vi "JKI_UI Console.vi"() -> ()   [LabVIEW 2017, in "UI Console_JKI.lvlib"]
uses:
  UI Console_JKI.lvlib
  <userlib>/_NEVSTOP/JKI State Machine ++/_Support/_Create Data Queue.vi
  <userlib>/_NEVSTOP/JKI State Machine ++/_Support/_JKISMQFGV.vi
  <userlib>/_NEVSTOP/JKI State Machine ++/JKI-State-Machine-Plus.lvlib
panel:
  in  "Error Simulator":bool
  in  "Transaction Enable Signal":bool
  in  "KeyPad Enable Signal":bool
  in  "Keypad":T1
  out "Keypad String":string
  in  "Card Reader Enable Signal":bool
  in  "Transactions":T2
  in  "Card Reader":bool
  out "State History":string
  in  "Name(\"\" to use uuid)":string="UI Console"
  # "KeyPad"
  # "Transaction"
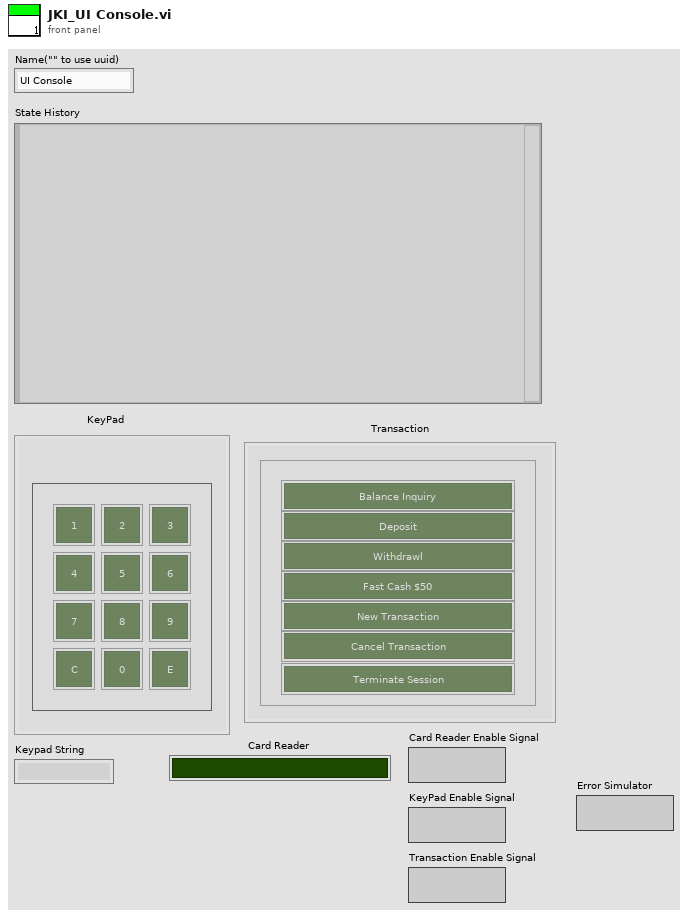
[diagram p1: front panel]
types:
  T1 = cluster{"Key":bool, "Key 2":bool, "Key 3":bool, "Key 4":bool, "Key 5":bool, "Key 6":bool, "Key 7":bool, "Key 8":bool, "Key 9":bool, "Key 10":bool, "Key 11":bool, "Key 12":bool}
  T2 = cluster{"xaction":bool, "xaction 2":bool, "xaction 3":bool, "xaction 4":bool, "xaction 5":bool, "xaction 6":bool, "xaction 7":bool}
  T3 = enum32{"Invalid", "Standard", "Closed", "Hidden", "Minimized", "Maximized"}
  T4 = enum32{"invalid app kind", "Development System", "Run Time System", "Student Edition", "Embedded LabVIEW", "Evaluation", "Custom"}
  T5 = enum8{"Enabled", "Disabled", "Disabled and Grayed Out"}
  T6 = cluster{"Core":cluster{"Current VI Reference":refnum<vi>, "Close Panel on Exit?":bool}, "Your Boolean data":bool, "New Character":i32, "Keypad String":string, "Transaction Type":i32}
  T7 = cluster{"Current VI Reference":refnum<vi>, "Close Panel on Exit?":bool}
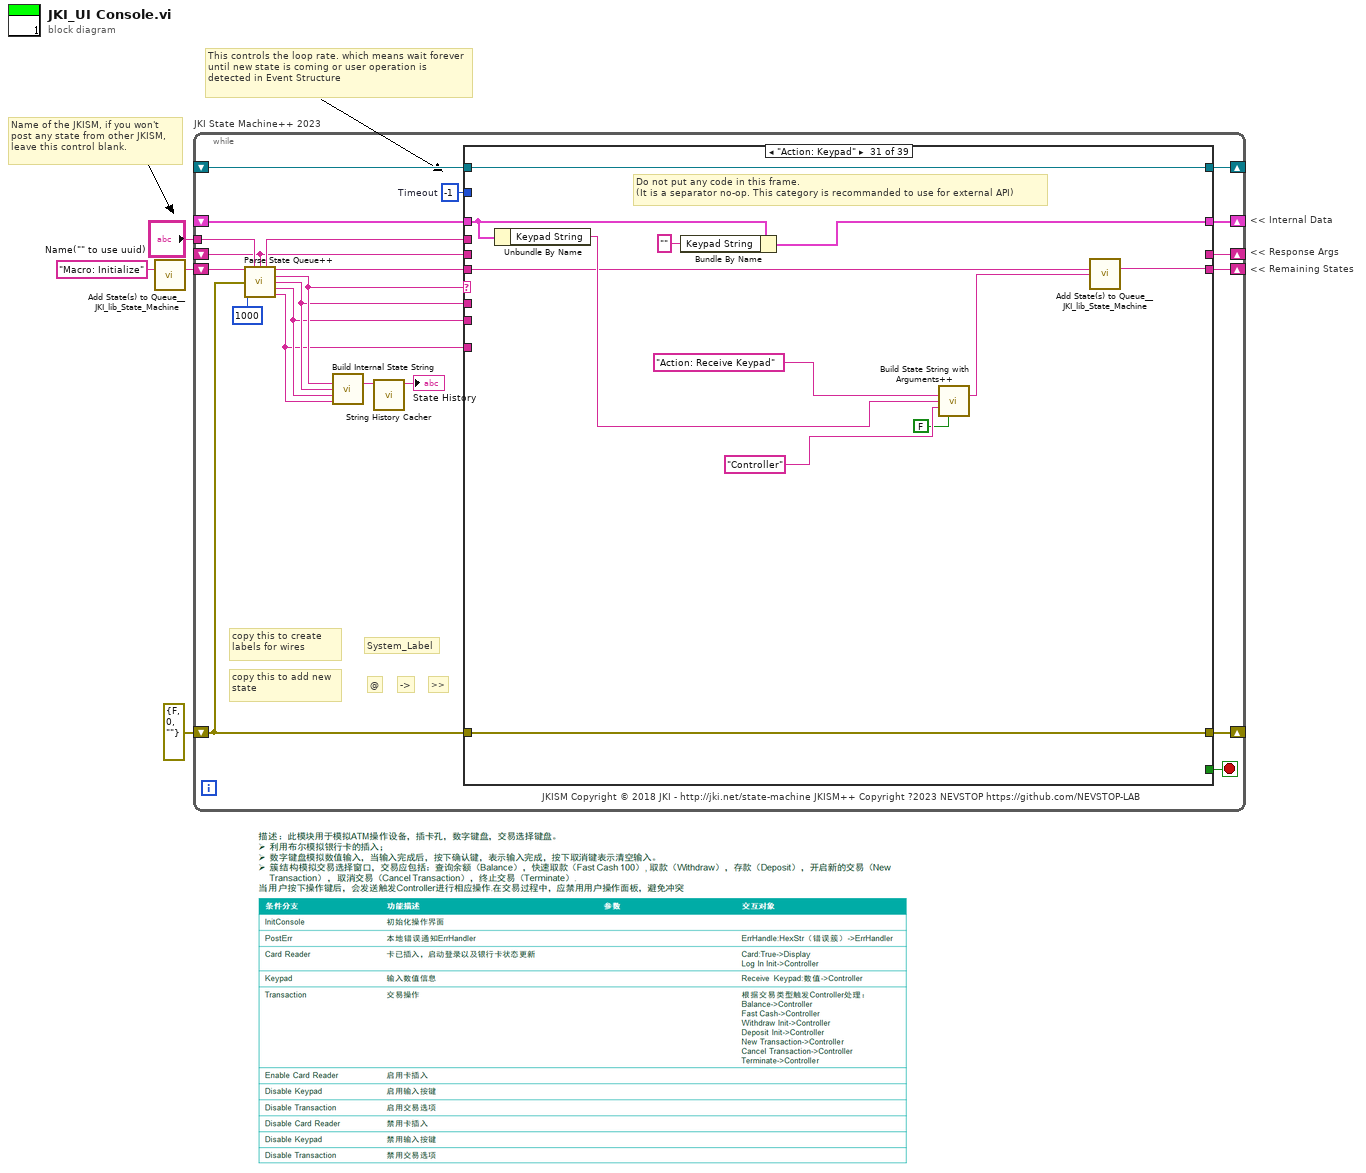
[diagram p0: block diagram]
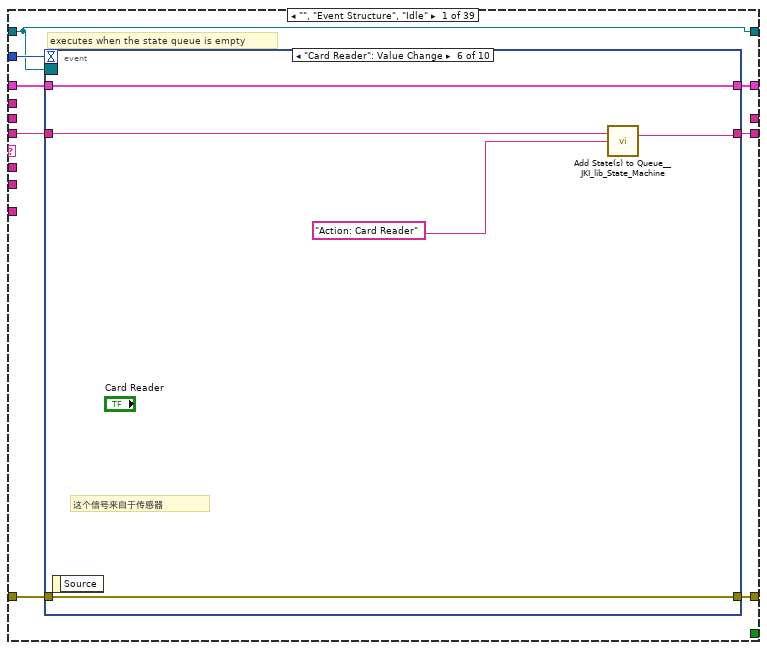
[diagram p2: hidden frame]
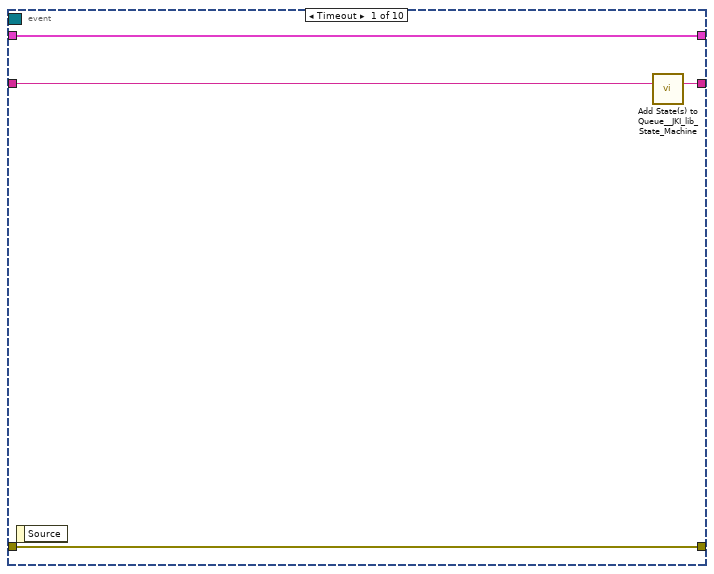
[diagram p3: hidden frame]
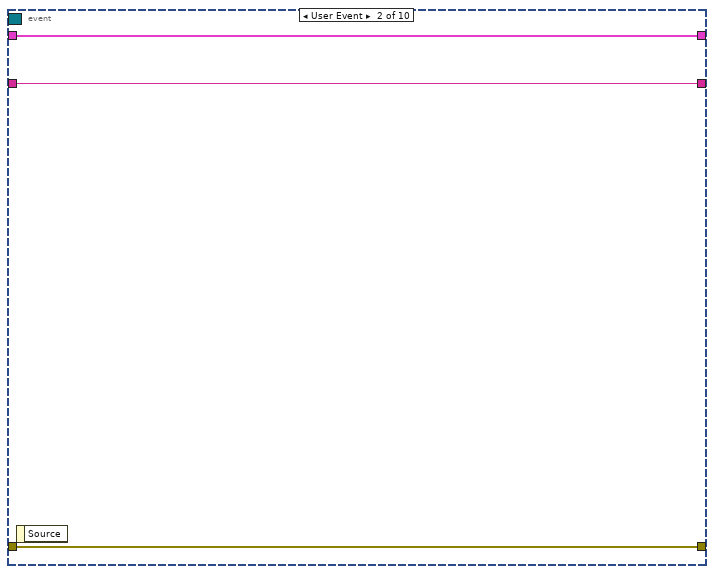
[diagram p4: hidden frame]
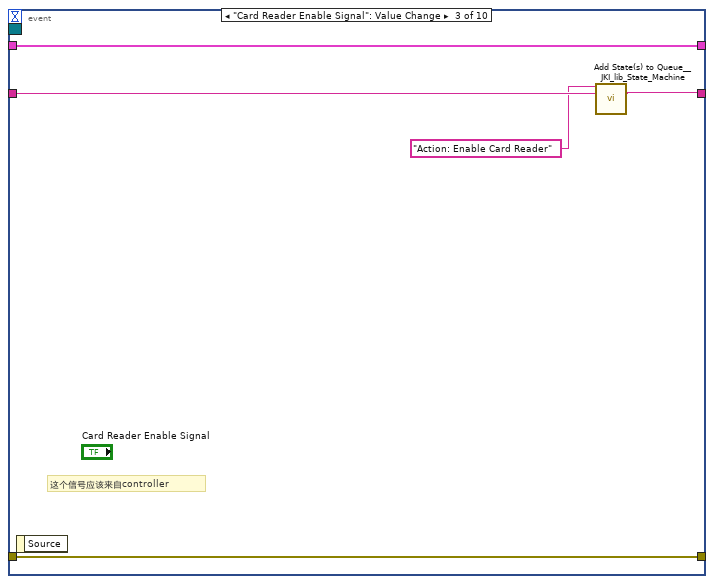
[diagram p5: hidden frame]
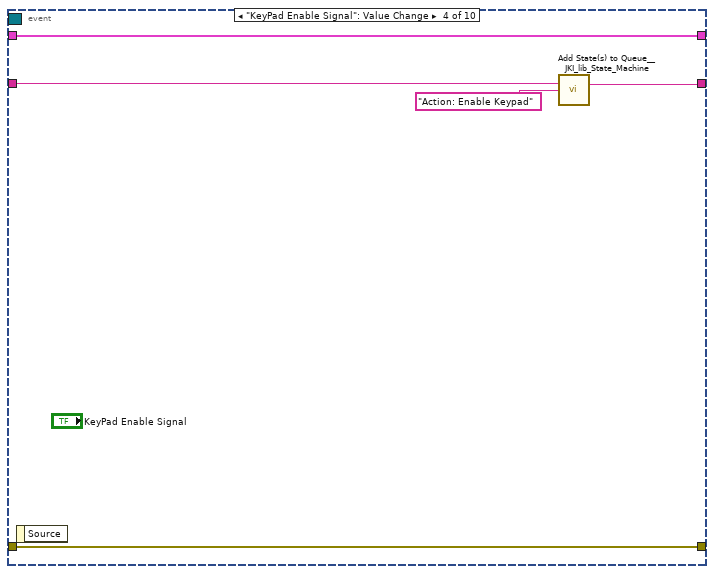
[diagram p6: hidden frame]
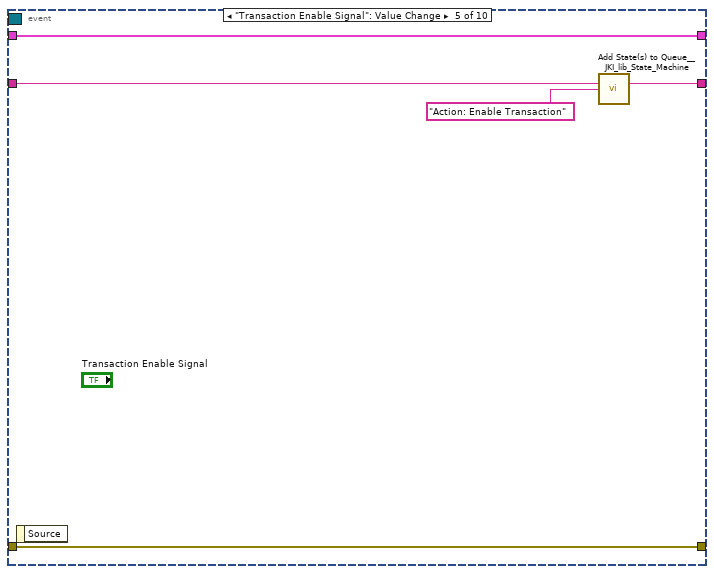
[diagram p7: hidden frame]
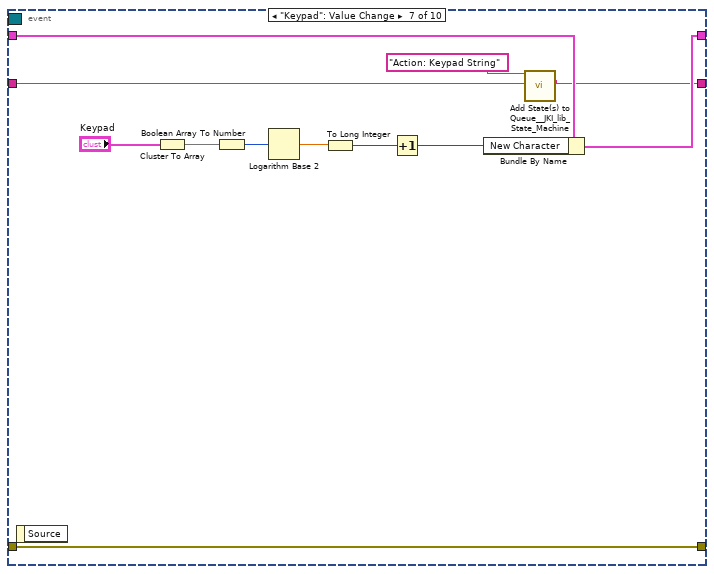
[diagram p8: hidden frame]
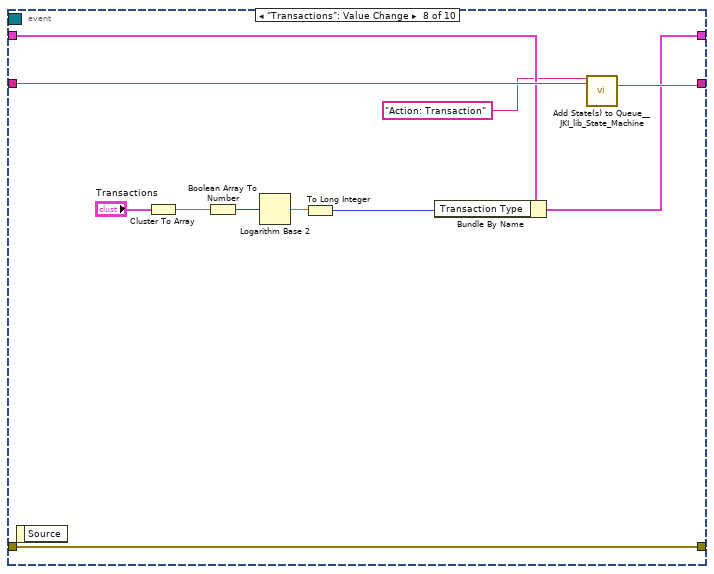
[diagram p9: hidden frame]
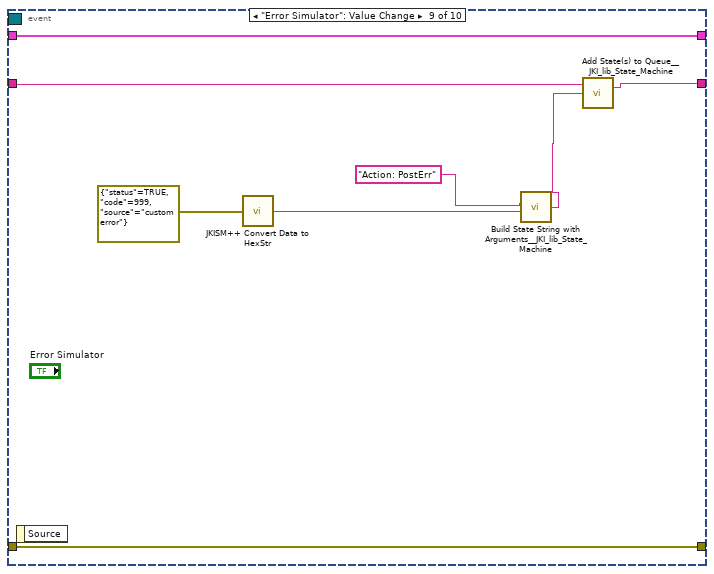
[diagram p10: hidden frame]
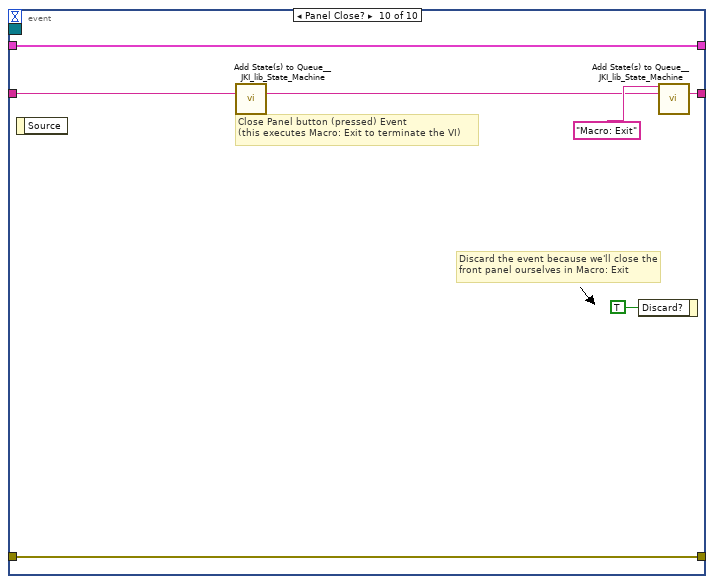
[diagram p11: hidden frame]
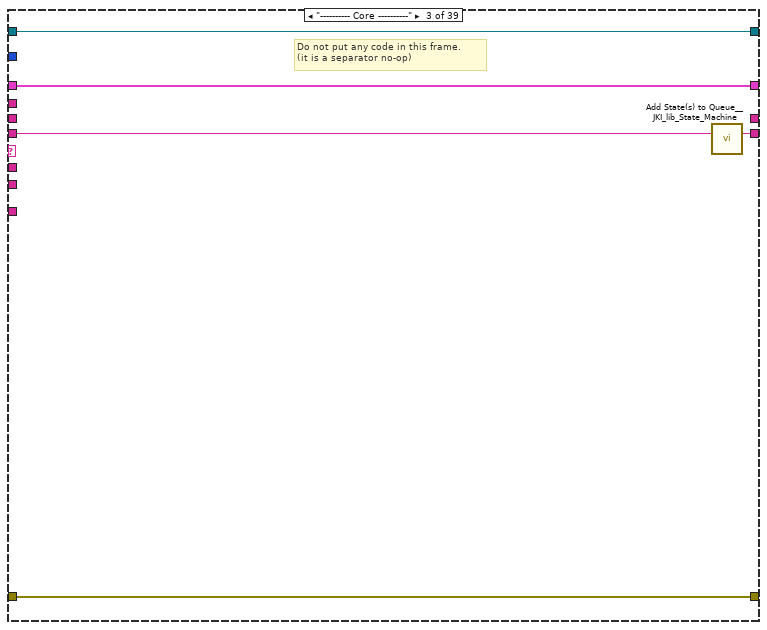
[diagram p13: hidden frame]
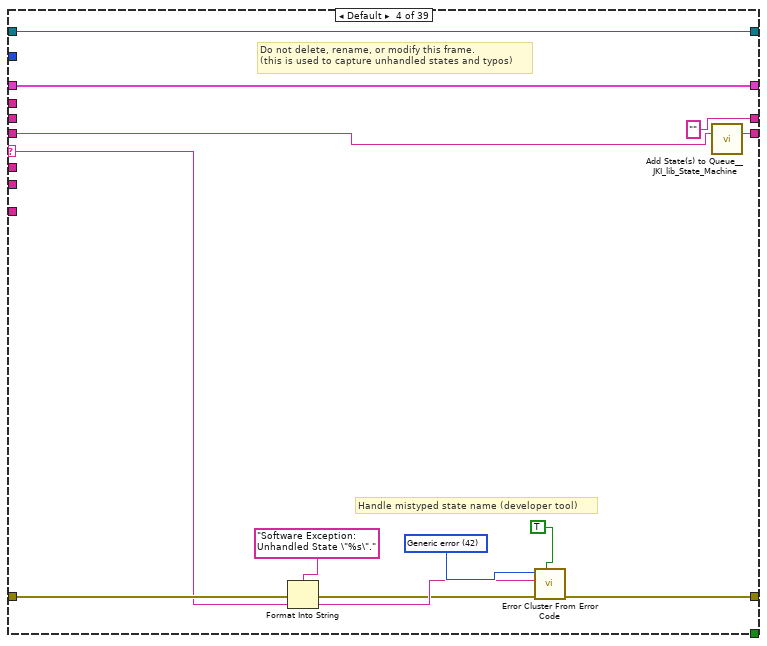
[diagram p14: hidden frame]
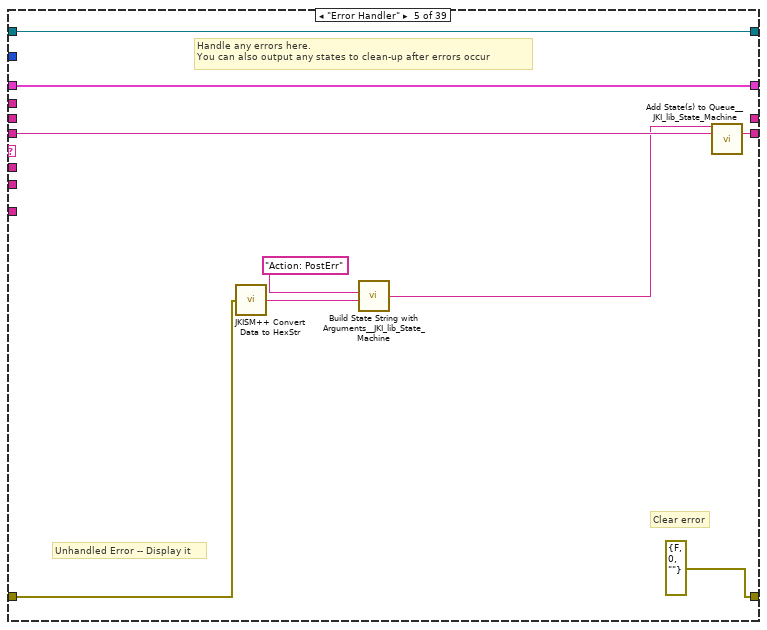
[diagram p15: hidden frame]
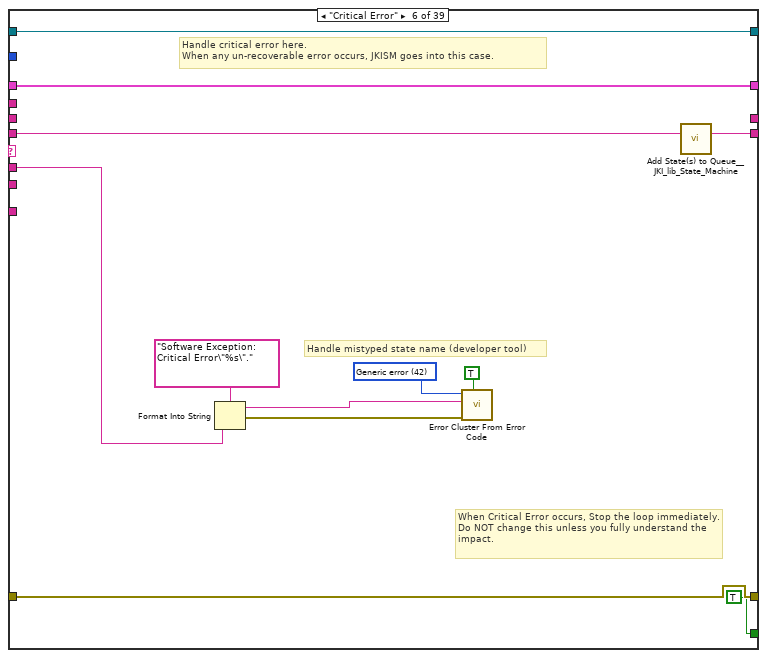
[diagram p16: hidden frame]
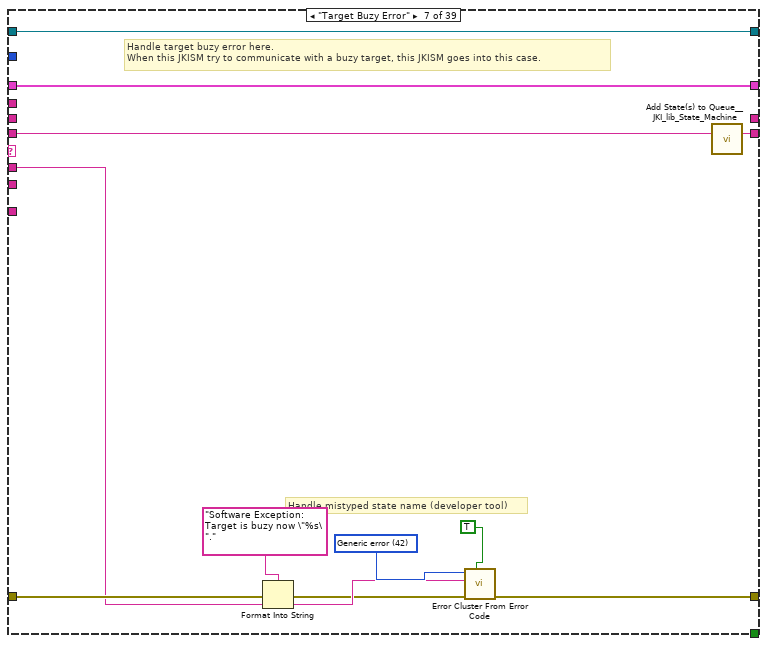
[diagram p17: hidden frame]
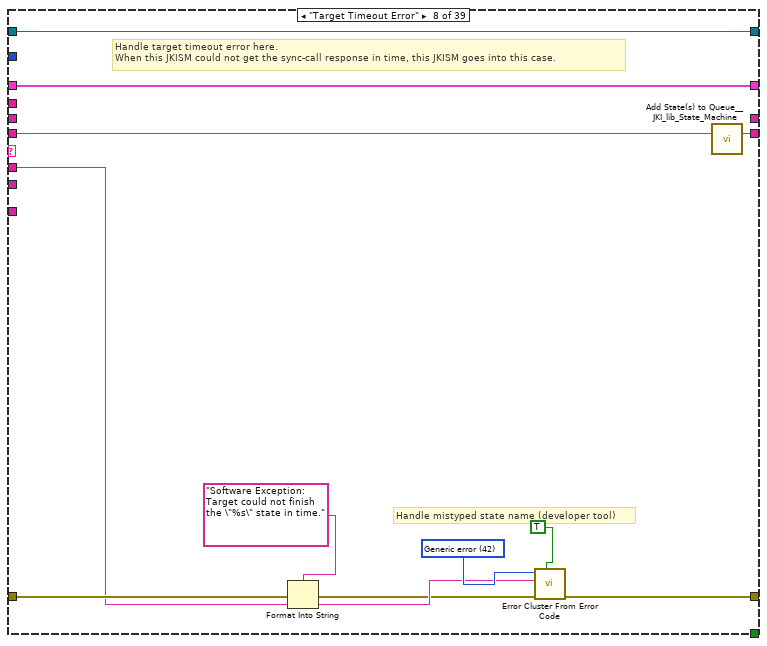
[diagram p18: hidden frame]
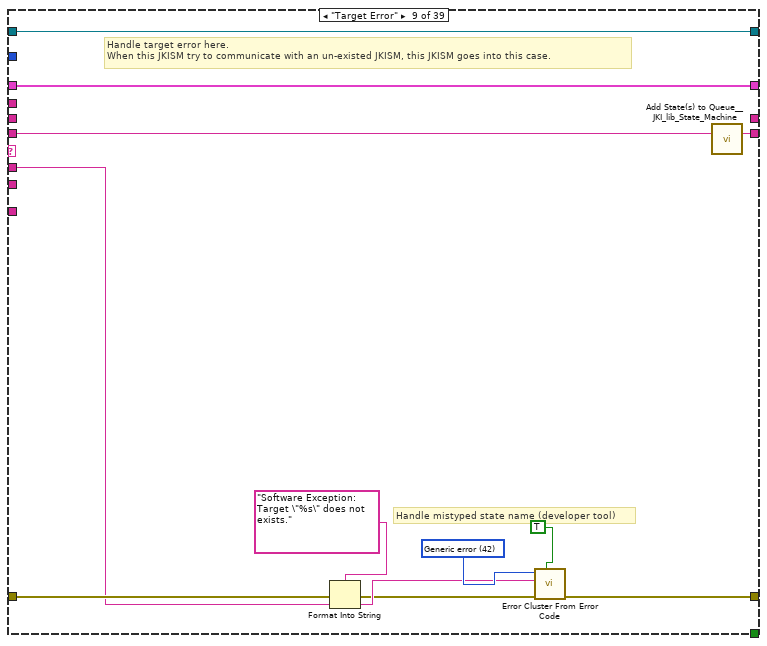
[diagram p19: hidden frame]
diagram:
  # "<< Internal Data"
  # "<< Response Args"
  # "<< Remaining States"
  # "Name of the JKISM, if you won't post any state from other JKISM,  leave this control blank."
  # "This controls the loop rate. which means wait forever until new state is coming or user operation is detected in Event Structure"
  n1 = call <vilib>:"Add State(s) to Queue__JKI_lib_State_Machine.vi"("State(s) in (\"\")"="Macro: Initialize") -> ("States Out"=w2:string)  [unwired: 14 in]
  n2 = while "JKI State Machine++ 2023" {
    shift-right: [w21] -> _
    shift-left: _ -> [w20]
    shift-right: [w24] -> _
    shift-left: errorcluster {"status"=FALSE, "code"=0, "source"=""} ("error out") -> [w18]
    shift-right: [w23] -> _
    shift-left: w2 -> [w25]
    tunnel: "Name(\"\" to use uuid)" -> [w13]
    shift-right: [w16] -> _
    shift-left: _ -> [w5]
    shift-right: [w15] -> _
    shift-left: _ -> [w14]
    stop <- w22 stop-if-true
    w19 = -1  # Timeout
    # "JKISM Copyright © 2018 JKI - http://jki.net/state-machine JKISM++ Copyright ?2023 NEVSTOP https://github.com/NEVSTOP-LAB"
    # "copy this to add new state"
    # ">>"
    # "->"
    # "@"
    # "copy this to create labels for wires"
    # "System_Label"
    n3 = call <userlib>:"Parse State Queue++.vi"("State Queue"=w25, "Name(\"\" to use uuid)"=w13, "Response Arguments"=w5, "Error In (no error)"=w18, "Response Timeout(5000ms)"=1000 ("Response Timeout(1000ms)")) -> ("Name Used"=w6:string, "Remaining States"=w26:string, "Current State"=w10:string, "Arguments"=w9:string, "Argument - State"=w8:string, "From Who"=w7:string)  [unwired: 5 in]
    n4 = call <userlib>:"Build Internal State String.vi"("State"=w10, "Arguments (\"\")"=w9, "Arg-State (\"\")"=w8, "Source (\"\")"=w7) -> ("State with Arguments"=w11:string)  [unwired: 11 in]
    n5 = call <userlib>:"String History Cacher.vi"("String"=w11) -> ("String Cache"=→"State History":string)  [unwired: 10 in]
    n6 = case shown="\"Action: Keypad\"" w10 {
      selector: w10 -> [_ _ _ w111 _ _ _ _ _ _ _ _ _ _ _ _ _ _ _ _ _ _ _ _ _ _ _ _ _ _ _ _ _ _ _ _ _ _ _]
      tunnel: w26 -> [w34 w102 w108 w115 w130 w140 w143 w160 w172 w181 w185 w200 w206 w211 w221 w228 w233 w239 w243 w249 w254 w261 w273 w343 w349 w360 w365 w377 w385 w401 w420 w430 w471 w491 w498 w505 w512 w519 w526]
      tunnel: w9 -> [_ _ _ _ _ w133 w145 w156 w168 _ _ _ _ _ _ _ _ _ _ _ _ w256 w267 _ _ _ _ _ w381 _ _ _ _ _ _ _ _ _ _]
      tunnel: w20 -> [w32 w101 w105 w113 w127 w141 w147 w158 w170 w180 w184 w193 w204 w208 _ w223 w230 w238 w242 w246 w252 w259 w269 w340 w346 w357 w362 w375 w387 w414 w417 w432 w465 w489 w496 w503 w510 w517 w524]
      tunnel: [w31 w103 w106 w117 errorcluster {"status"=FALSE, "code"=0, "source"=""} ("error out") w142 w150 w162 w174 w182 w186 w197 w203 w209 w218 w224 w231 w234 w241 w247 w251 w257 w270 w341 w347 w358 w363 w369 w379 w407 w425 w427 w469 w485 w492 w499 w506 w513 w520] -> w24
      tunnel: w18 -> [w30 w103 w106 w116 w123 w142 w149 w161 w173 w182 w186 w197 w203 w209 w218 w225 w231 _ w244 w247 w251 w258 w271 w341 w347 w358 w363 w367 w380 w407 w425 w427 w469 w486 w493 w500 w507 w514 w521]
      tunnel: [w33 w102 w107 w114 w129 w139 w148 w159 w171 w181 w185 w199 w205 w210 w220 w227 w232 w239 w243 w248 w253 w260 w272 w342 w348 w359 w364 w376 w384 w400 w419 w429 w470 w490 w497 w504 w511 w518 w525] -> w23
      tunnel: [_ _ _ _ _ TRUE _ _ _ _ _ _ TRUE _ _ _ _ _ _ _ _ _ _ _ _ _ _ _ _ _ _ _ _ _ _ _ _ _ _] -> w22
      tunnel: [w29 w101 w105 w113 w127 w141 w147 w158 w170 w180 w184 w198 w204 w208 w219 w223 w230 w238 w242 w246 w252 w259 w269 w340 w346 w357 w362 w375 w387 w414 w415 w432 w464 w489 w496 w503 w510 w517 w524] -> w21
      tunnel: w19 -> [w28 _ _ _ _ _ _ _ _ _ _ _ _ _ _ _ _ _ _ _ _ _ _ _ _ _ _ _ _ _ _ _ _ _ _ _ _ _ _]
      tunnel: w7 -> [_ _ _ _ _ _ _ _ _ _ _ _ _ _ _ _ _ _ _ _ _ _ _ _ _ _ _ _ _ _ _ _ _ _ _ _ _ _ _]
      tunnel: w8 -> [_ _ _ _ _ _ _ _ _ _ _ _ _ _ _ _ _ _ _ _ _ _ _ _ _ _ _ _ _ _ _ _ _ _ _ _ _ _ _]
      tunnel: [_ _ _ "" _ _ _ _ _ _ _ _ _ _ _ _ _ _ _ _ _ _ _ _ _ _ _ _ _ _ _ _ w462 _ _ _ _ _ _] -> w16
      tunnel: [w27 w100 w104 w109 w126 w131 w144 w155 w167 w179 w183 w187 w201 w207 w215 w222 w229 w237 w240 w245 w250 w255 w266 w339 w344 w350 w361 w374 w386 w413 w426 w433 w468 w488 w495 w502 w509 w516 w523] -> w15
      tunnel: w14 -> [w27 w100 w104 w109 w126 w131 w144 w155 w167 w179 w183 w187 w201 w207 w215 w222 w229 _ w240 w245 w250 w255 w266 w339 w344 w350 w361 w374 w386 w413 w426 w433 w468 w488 w495 w502 w509 w516 w523]
      tunnel: w6 -> [_ _ _ _ _ _ _ _ _ _ _ _ _ _ _ _ _ w236 _ _ _ _ _ _ _ _ _ _ _ _ _ _ _ _ _ _ _ _ _]
      tunnel: w5 -> [_ _ _ _ _ _ _ _ _ _ _ _ _ _ _ _ _ _ _ _ _ _ _ _ _ _ _ _ _ _ _ _ _ _ _ _ _ _ _]
      frame "", "Event Structure", "Idle" {
        # "executes when the state queue is empty"
        n7 = event shown="[5] \"Card Reader\": Value Change" {
          selector: w27 -> [_ _ _ _ _ _ _ _ _ _]
          dyn-events: _ -> [_ _ _ _ _ _ _ _ _ _]
          timeout: w28 -> [_ _ _ _ _ _ _ _ _ _]
          tunnel: w34 -> [w38 w41 w45 w49 w54 w59 w68 w79 w87 w93]
          tunnel: [w37 w41 w44 w48 w53 w58 w67 w78 w86 w99] -> w33
          tunnel: w32 -> [w35 w39 w46 w50 w55 w61 w71 w77 w91 w97]
          tunnel: [w36 w40 w43 w51 w56 w60 w73 w84 w92 w98] -> w31
          tunnel: w30 -> [w36 w40 w43 w51 w56 w60 w73 w84 w92 w98]
          tunnel: [w35 w39 w46 w50 w55 w61 w70 w75 w91 w97] -> w29
          event Timeout {
            n8 = event-data() -> ()  [unwired: 1 in, 1 out]
            n9 = call <vilib>:"Add State(s) to Queue__JKI_lib_State_Machine.vi"("State(s) in (\"\")"=w38) -> ("States Out"=w37:string)  [unwired: 14 in]
          }
          event User Event {
            n10 = event-data() -> ()  [unwired: 1 in, 1 out]
          }
          event "Card Reader Enable Signal": Value Change {
            # "这个信号应该来自controller"
            n11 = event-data() -> ()  [unwired: 1 in, 1 out]
            n12 = call <vilib>:"Add State(s) to Queue__JKI_lib_State_Machine.vi"("State(s) in Front (\"\")"="Action: Enable Card Reader", "State(s) in (\"\")"=w45) -> ("States Out"=w44:string)  [unwired: 13 in]
          }
          event "KeyPad Enable Signal": Value Change {
            n13 = event-data() -> ()  [unwired: 1 in, 1 out]
            n14 = call <vilib>:"Add State(s) to Queue__JKI_lib_State_Machine.vi"("State(s) in (\"\")"=w49, "State(s) at Back (\"\")"="Action: Enable Keypad" ("State(s) at Back (\"\")")) -> ("States Out"=w48:string)  [unwired: 13 in]
          }
          event "Transaction Enable Signal": Value Change {
            n15 = event-data() -> ()  [unwired: 1 in, 1 out]
            n16 = call <vilib>:"Add State(s) to Queue__JKI_lib_State_Machine.vi"("State(s) in (\"\")"=w54, "State(s) at Back (\"\")"="Action: Enable Transaction" ("State(s) at Back (\"\")")) -> ("States Out"=w53:string)  [unwired: 13 in]
          }
          event "Card Reader": Value Change {
            # "这个信号来自于传感器"
            n17 = event-data() -> ()  [unwired: 1 in, 1 out]
            n18 = call <vilib>:"Add State(s) to Queue__JKI_lib_State_Machine.vi"("State(s) in (\"\")"=w59, "State(s) at Back (\"\")"="Action: Card Reader") -> ("States Out"=w58:string)  [unwired: 13 in]
          }
          event "Keypad": Value Change {
            n19 = event-data() -> ()  [unwired: 1 in, 1 out]
            n20 = Cluster To Array(cluster="Keypad") -> (array=w64:bool[])
            n21 = Boolean Array To Number(Boolean array=w64) -> (number=w72:u32)
            n22 = Logarithm Base 2(1:w72) -> (0:w69:dbl)
            n23 = To Long Integer(number=w69) -> (32bit integer=w63:i32)
            n24 = Increment(x=w63) -> (x+1=w62:i32)
            n25 = Bundle By Name(cluster=w71, "New Character"=w62) -> (w70:T6)
            n26 = call <vilib>:"Add State(s) to Queue__JKI_lib_State_Machine.vi"("State(s) in Front (\"\")"="Action: Keypad String" ("State(s) in Front (\"\")"), "State(s) in (\"\")"=w68) -> ("States Out"=w67:string)  [unwired: 13 in]
          }
          event "Transactions": Value Change {
            n27 = event-data() -> ()  [unwired: 1 in, 1 out]
            n28 = Cluster To Array(cluster="Transactions") -> (array=w81:bool[])
            n29 = Boolean Array To Number(Boolean array=w81) -> (number=w83:u32)
            n30 = Logarithm Base 2(1:w83) -> (0:w82:dbl)
            n31 = To Long Integer(number=w82) -> (32bit integer=w76:i32)
            n32 = Bundle By Name(cluster=w77, "Transaction Type"=w76) -> (w75:T6)
            n33 = call <vilib>:"Add State(s) to Queue__JKI_lib_State_Machine.vi"("State(s) in Front (\"\")"="Action: Transaction" ("State(s) in Front (\"\")"), "State(s) in (\"\")"=w79) -> ("States Out"=w78:string)  [unwired: 13 in]
          }
          event "Error Simulator": Value Change {
            n34 = event-data() -> ()  [unwired: 1 in, 1 out]
            n35 = call <userlib>:"JKISM++ Convert Data to HexStr.vi"("Variant"=errorcluster {"status"=TRUE, "code"=999, "source"="custom error"} ("error in (no error)")) -> ("HEX String (0-9,A-F)"=w89:string)  [unwired: 8 in]
            n36 = call <vilib>:"Build State String with Arguments__JKI_lib_State_Machine.vi"("Arguments (\"\")"=w89, "State"="Action: PostErr" ("States")) -> ("State with Arguments"=w88:string)  [unwired: 4 in]
            n37 = call <vilib>:"Add State(s) to Queue__JKI_lib_State_Machine.vi"("State(s) in (\"\")"=w87, "State(s) at Back (\"\")"=w88) -> ("States Out"=w86:string)  [unwired: 13 in]
          }
          event Panel Close? {
            # "Discard the event because we'll close the front panel ourselves in Macro: Exit"
            # "Close Panel button (pressed) Event\n(this executes Macro: Exit to terminate the VI)"
            n38 = event-data() -> ()  [unwired: 1 in, 1 out]
            n39 = call <vilib>:"Add State(s) to Queue__JKI_lib_State_Machine.vi"("State(s) in (\"\")"=w93) -> ("States Out"=w94:string)  [unwired: 14 in]
            n40 = event-data("Discard?"=TRUE) -> ()  [unwired: 1 in, 1 out]
            n41 = call <vilib>:"Add State(s) to Queue__JKI_lib_State_Machine.vi"("State(s) in Front (\"\")"="Macro: Exit", "State(s) in (\"\")"=w94) -> ("States Out"=w99:string)  [unwired: 13 in]
          }
        }
      }
      frame "JKISM++ Documentation" {
        # "JKISM++ Documentation"
        # "State Syntax:\nStateCategory: State >> Argument @|-> JKISMName\nLine Terminator: Line feed\n\nExample:\nUI: Help >> About @Main\nUI: Help >> About ->Main"
        # "Commenting:\nTo add a comment use \"//\" or \"#\" and all text to the right will be ignored\nCommenting Example:\nUI: Initialize // This initializes the UI\n# This whole line is a comment\n// Another comment line"
        # "Where \"UI\" is the state category\nWhere \"Help\" is the state\nWhere \"About\" is the argument\nWhere \"Main\" is the Name of JKISM,which actually run the \"UI: Help >> About\"\n\n    \"@\" stands for sync state. Current JKISM will wait until the state is finished. \n            - if \"Main\" named JKISM does not exist, \"Target Error\" will occur.\n            - if \"Main\" named JKISM is in another sync remote state, \"Target Buzy Error\" will occur.\n            - if \"Main\" named JKISM could not finish the state in time, \"Target Timeout Error\" will occur.\n            - if everything is right. \"Response\" will occur with Argument back from \"Main\" named JKISM. \n\n    \"->\" stands for async state. Current JKISM will post the state and continue to next state in next iteration.\n            - if \"Main\" named JKISM does not exist, \"Target Error\" will occur.\n            - if everything is right. \"Async Message Posted\" will occur.\n            - After State is finished. Caller will receive a \"Async Response\" state from callee.\n\nWhen duplicated name is used for multiple JKISM module or some framework problem happens, \"Critical Error\" will occur."
      }
      frame "---------- Core ----------" {
        # "Do not put any code in this frame.\n(it is a separator no-op)"
        n42 = call <vilib>:"Add State(s) to Queue__JKI_lib_State_Machine.vi"("State(s) in (\"\")"=w108) -> ("States Out"=w107:string)  [unwired: 14 in]
      }
      frame Default {
        w120 = 42 items=["No error", "Argument error", "Memory is full", "Out of zone", "End of file", "File already open", "Generic file I/O error", "File not found", "File permission error", "Disk is full", "Duplicate path", "Too many files open", "System feature not enabled", "Resource file not found", "Cannot add resource", "Resource not found", "Image not found", "Image memory error", "Pen does not exist", "Config type invalid", "Config token not found", "Config parse error", "Config memory error", "Bad external code format", "Bad external code offset", "External code not present", "Null window", "Destroy window error", "Null menu", "Print aborted", "Bad print record", "Print driver error", "Windows error during printing", "Memory error during printing", "Print dialog error", "Generic print error", "Invalid device refnum", "Device not found", "Device parameter error", "Device unit error", "Cannot open device", "Device call aborted", "Generic error", "Cancelled by user", "Object ID too low", "Object ID too high", "Object not in heap", "Unknown heap", "Unknown object (invalid DefProc)", "Unknown object (DefProc not in table)", "Message out of range", "Invalid (null) method", "Unknown message", "Manager call not supported", "Bad address", "Network operation in progress", "Network operation timed out", "Connection is busy", "Network attribute not supported", "Network error", "Address in use", "System out of memory", "Connection aborted", "Connection refused", "Not connected", "Already connected", "Connection closed", "Initialization error (interapplication manager)", "Bad occurrence", "Wait on unbound occurrence handler", "Occurrence queue overflow", "Datalog type conflict", "Unused", "Unrecognized type (interapplication manager)", "Memory corrupt", "Failed to make temporary DLL", "Old CIN version", "Drag socket not found", "Failed to load drop-object", "Failed to register OLE object", "Failed to release OLE object", "Format specifier type mismatch", "Unknown format specifier", "Too few format specifiers", "Too many format specifiers", "Scan failed", "Newer CIN version", "Error converting to variant", "Runtime menu error", "Password tampered", "Variant attribute not found", "Incompatible variant data type", "Event data is not available", "Event Store is not present", "Occurrence is not found", "Event Queue is not created", "Event info is not available", "Refnum passed is NULL", "Error retrieving Class GUID", "Error retrieving CoClass GUID", "Error retrieving TypeLib GUID.", "Bad built application magic bytes.", "Specific driver is different from the specific driver associated with the Logical Name.", "There is no session opened to the class driver.", "Max Error", "MAX - Error with config objects", "MAX - Error loading configuration", "MAX - Group not supported"]
        # "Do not delete, rename, or modify this frame.\n(this is used to capture unhandled states and typos)"
        # "Handle mistyped state name (developer tool)"
        n43 = Format Into String(format string="Software Exception: Unhandled State \"%s\"." ("message"), error in=w116, w111) -> (resulting string=w119:string, error out=w118:errorcluster)  [unwired: 1 in]
        n44 = call <vilib>:"Error Cluster From Error Code.vi"("show call chain? (False)"=TRUE, "error in (no error)"=w118, "error message (\"\")"=w119, "error code (0)"=w120) -> ("error out"=w117:errorcluster)  [unwired: 5 in]
        n45 = call <vilib>:"Add State(s) to Queue__JKI_lib_State_Machine.vi"("State(s) in (\"\")"=w115) -> ("States Out"=w114:string)  [unwired: 14 in]
      }
      frame "Error Handler" {
        # "Unhandled Error -- Display it"
        # "Handle any errors here.\nYou can also output any states to clean-up after errors occur"
        # "Clear error"
        n46 = call <userlib>:"JKISM++ Convert Data to HexStr.vi"("Variant"=w123) -> ("HEX String (0-9,A-F)"=w125:string)  [unwired: 8 in]
        n47 = call <vilib>:"Build State String with Arguments__JKI_lib_State_Machine.vi"("Arguments (\"\")"=w125, "State"="Action: PostErr") -> ("State with Arguments"=w122:string)  [unwired: 4 in]
        n48 = call <vilib>:"Add State(s) to Queue__JKI_lib_State_Machine.vi"("State(s) in Front (\"\")"=w122, "State(s) in (\"\")"=w130) -> ("States Out"=w129:string)  [unwired: 13 in]
      }
      frame "Critical Error" {
        w137 = 42 items=["No error", "Argument error", "Memory is full", "Out of zone", "End of file", "File already open", "Generic file I/O error", "File not found", "File permission error", "Disk is full", "Duplicate path", "Too many files open", "System feature not enabled", "Resource file not found", "Cannot add resource", "Resource not found", "Image not found", "Image memory error", "Pen does not exist", "Config type invalid", "Config token not found", "Config parse error", "Config memory error", "Bad external code format", "Bad external code offset", "External code not present", "Null window", "Destroy window error", "Null menu", "Print aborted", "Bad print record", "Print driver error", "Windows error during printing", "Memory error during printing", "Print dialog error", "Generic print error", "Invalid device refnum", "Device not found", "Device parameter error", "Device unit error", "Cannot open device", "Device call aborted", "Generic error", "Cancelled by user", "Object ID too low", "Object ID too high", "Object not in heap", "Unknown heap", "Unknown object (invalid DefProc)", "Unknown object (DefProc not in table)", "Message out of range", "Invalid (null) method", "Unknown message", "Manager call not supported", "Bad address", "Network operation in progress", "Network operation timed out", "Connection is busy", "Network attribute not supported", "Network error", "Address in use", "System out of memory", "Connection aborted", "Connection refused", "Not connected", "Already connected", "Connection closed", "Initialization error (interapplication manager)", "Bad occurrence", "Wait on unbound occurrence handler", "Occurrence queue overflow", "Datalog type conflict", "Unused", "Unrecognized type (interapplication manager)", "Memory corrupt", "Failed to make temporary DLL", "Old CIN version", "Drag socket not found", "Failed to load drop-object", "Failed to register OLE object", "Failed to release OLE object", "Format specifier type mismatch", "Unknown format specifier", "Too few format specifiers", "Too many format specifiers", "Scan failed", "Newer CIN version", "Error converting to variant", "Runtime menu error", "Password tampered", "Variant attribute not found", "Incompatible variant data type", "Event data is not available", "Event Store is not present", "Occurrence is not found", "Event Queue is not created", "Event info is not available", "Refnum passed is NULL", "Error retrieving Class GUID", "Error retrieving CoClass GUID", "Error retrieving TypeLib GUID.", "Bad built application magic bytes.", "Specific driver is different from the specific driver associated with the Logical Name.", "There is no session opened to the class driver.", "Max Error", "MAX - Error with config objects", "MAX - Error loading configuration", "MAX - Group not supported"]
        # "Handle critical error here.\nWhen any un-recoverable error occurs, JKISM goes into this case."
        # "When Critical Error occurs, Stop the loop immediately. Do NOT change this unless you fully understand the impact."
        # "Handle mistyped state name (developer tool)"
        n49 = Format Into String(format string="Software Exception: Critical Error\"%s\"." ("message"), w133) -> (resulting string=w136:string, error out=w135:errorcluster)  [unwired: 2 in]
        n50 = call <vilib>:"Error Cluster From Error Code.vi"("show call chain? (False)"=TRUE, "error in (no error)"=w135, "error message (\"\")"=w136, "error code (0)"=w137) -> ()  [unwired: 5 in, 1 out]
        n51 = call <vilib>:"Add State(s) to Queue__JKI_lib_State_Machine.vi"("State(s) in (\"\")"=w140) -> ("States Out"=w139:string)  [unwired: 14 in]
      }
      frame "Target Buzy Error" {
        w153 = 42 items=["No error", "Argument error", "Memory is full", "Out of zone", "End of file", "File already open", "Generic file I/O error", "File not found", "File permission error", "Disk is full", "Duplicate path", "Too many files open", "System feature not enabled", "Resource file not found", "Cannot add resource", "Resource not found", "Image not found", "Image memory error", "Pen does not exist", "Config type invalid", "Config token not found", "Config parse error", "Config memory error", "Bad external code format", "Bad external code offset", "External code not present", "Null window", "Destroy window error", "Null menu", "Print aborted", "Bad print record", "Print driver error", "Windows error during printing", "Memory error during printing", "Print dialog error", "Generic print error", "Invalid device refnum", "Device not found", "Device parameter error", "Device unit error", "Cannot open device", "Device call aborted", "Generic error", "Cancelled by user", "Object ID too low", "Object ID too high", "Object not in heap", "Unknown heap", "Unknown object (invalid DefProc)", "Unknown object (DefProc not in table)", "Message out of range", "Invalid (null) method", "Unknown message", "Manager call not supported", "Bad address", "Network operation in progress", "Network operation timed out", "Connection is busy", "Network attribute not supported", "Network error", "Address in use", "System out of memory", "Connection aborted", "Connection refused", "Not connected", "Already connected", "Connection closed", "Initialization error (interapplication manager)", "Bad occurrence", "Wait on unbound occurrence handler", "Occurrence queue overflow", "Datalog type conflict", "Unused", "Unrecognized type (interapplication manager)", "Memory corrupt", "Failed to make temporary DLL", "Old CIN version", "Drag socket not found", "Failed to load drop-object", "Failed to register OLE object", "Failed to release OLE object", "Format specifier type mismatch", "Unknown format specifier", "Too few format specifiers", "Too many format specifiers", "Scan failed", "Newer CIN version", "Error converting to variant", "Runtime menu error", "Password tampered", "Variant attribute not found", "Incompatible variant data type", "Event data is not available", "Event Store is not present", "Occurrence is not found", "Event Queue is not created", "Event info is not available", "Refnum passed is NULL", "Error retrieving Class GUID", "Error retrieving CoClass GUID", "Error retrieving TypeLib GUID.", "Bad built application magic bytes.", "Specific driver is different from the specific driver associated with the Logical Name.", "There is no session opened to the class driver.", "Max Error", "MAX - Error with config objects", "MAX - Error loading configuration", "MAX - Group not supported"]
        # "Handle target buzy error here.\nWhen this JKISM try to communicate with a buzy target, this JKISM goes into this case."
        # "Handle mistyped state name (developer tool)"
        n52 = Format Into String(format string="Software Exception: Target is buzy now \"%s\"." ("message"), error in=w149, w145) -> (resulting string=w152:string, error out=w151:errorcluster)  [unwired: 1 in]
        n53 = call <vilib>:"Error Cluster From Error Code.vi"("show call chain? (False)"=TRUE, "error in (no error)"=w151, "error message (\"\")"=w152, "error code (0)"=w153) -> ("error out"=w150:errorcluster)  [unwired: 5 in]
        n54 = call <vilib>:"Add State(s) to Queue__JKI_lib_State_Machine.vi"("State(s) in (\"\")"=w143) -> ("States Out"=w148:string)  [unwired: 14 in]
      }
      frame "Target Timeout Error" {
        w165 = 42 items=["No error", "Argument error", "Memory is full", "Out of zone", "End of file", "File already open", "Generic file I/O error", "File not found", "File permission error", "Disk is full", "Duplicate path", "Too many files open", "System feature not enabled", "Resource file not found", "Cannot add resource", "Resource not found", "Image not found", "Image memory error", "Pen does not exist", "Config type invalid", "Config token not found", "Config parse error", "Config memory error", "Bad external code format", "Bad external code offset", "External code not present", "Null window", "Destroy window error", "Null menu", "Print aborted", "Bad print record", "Print driver error", "Windows error during printing", "Memory error during printing", "Print dialog error", "Generic print error", "Invalid device refnum", "Device not found", "Device parameter error", "Device unit error", "Cannot open device", "Device call aborted", "Generic error", "Cancelled by user", "Object ID too low", "Object ID too high", "Object not in heap", "Unknown heap", "Unknown object (invalid DefProc)", "Unknown object (DefProc not in table)", "Message out of range", "Invalid (null) method", "Unknown message", "Manager call not supported", "Bad address", "Network operation in progress", "Network operation timed out", "Connection is busy", "Network attribute not supported", "Network error", "Address in use", "System out of memory", "Connection aborted", "Connection refused", "Not connected", "Already connected", "Connection closed", "Initialization error (interapplication manager)", "Bad occurrence", "Wait on unbound occurrence handler", "Occurrence queue overflow", "Datalog type conflict", "Unused", "Unrecognized type (interapplication manager)", "Memory corrupt", "Failed to make temporary DLL", "Old CIN version", "Drag socket not found", "Failed to load drop-object", "Failed to register OLE object", "Failed to release OLE object", "Format specifier type mismatch", "Unknown format specifier", "Too few format specifiers", "Too many format specifiers", "Scan failed", "Newer CIN version", "Error converting to variant", "Runtime menu error", "Password tampered", "Variant attribute not found", "Incompatible variant data type", "Event data is not available", "Event Store is not present", "Occurrence is not found", "Event Queue is not created", "Event info is not available", "Refnum passed is NULL", "Error retrieving Class GUID", "Error retrieving CoClass GUID", "Error retrieving TypeLib GUID.", "Bad built application magic bytes.", "Specific driver is different from the specific driver associated with the Logical Name.", "There is no session opened to the class driver.", "Max Error", "MAX - Error with config objects", "MAX - Error loading configuration", "MAX - Group not supported"]
        # "Handle target timeout error here.\nWhen this JKISM could not get the sync-call response in time, this JKISM goes into this case."
        # "Handle mistyped state name (developer tool)"
        n55 = Format Into String(format string="Software Exception: Target could not finish the \"%s\" state in time." ("message"), error in=w161, w156) -> (resulting string=w164:string, error out=w163:errorcluster)  [unwired: 1 in]
        n56 = call <vilib>:"Error Cluster From Error Code.vi"("show call chain? (False)"=TRUE, "error in (no error)"=w163, "error message (\"\")"=w164, "error code (0)"=w165) -> ("error out"=w162:errorcluster)  [unwired: 5 in]
        n57 = call <vilib>:"Add State(s) to Queue__JKI_lib_State_Machine.vi"("State(s) in (\"\")"=w160) -> ("States Out"=w159:string)  [unwired: 14 in]
      }
      frame "Target Error" {
        w177 = 42 items=["No error", "Argument error", "Memory is full", "Out of zone", "End of file", "File already open", "Generic file I/O error", "File not found", "File permission error", "Disk is full", "Duplicate path", "Too many files open", "System feature not enabled", "Resource file not found", "Cannot add resource", "Resource not found", "Image not found", "Image memory error", "Pen does not exist", "Config type invalid", "Config token not found", "Config parse error", "Config memory error", "Bad external code format", "Bad external code offset", "External code not present", "Null window", "Destroy window error", "Null menu", "Print aborted", "Bad print record", "Print driver error", "Windows error during printing", "Memory error during printing", "Print dialog error", "Generic print error", "Invalid device refnum", "Device not found", "Device parameter error", "Device unit error", "Cannot open device", "Device call aborted", "Generic error", "Cancelled by user", "Object ID too low", "Object ID too high", "Object not in heap", "Unknown heap", "Unknown object (invalid DefProc)", "Unknown object (DefProc not in table)", "Message out of range", "Invalid (null) method", "Unknown message", "Manager call not supported", "Bad address", "Network operation in progress", "Network operation timed out", "Connection is busy", "Network attribute not supported", "Network error", "Address in use", "System out of memory", "Connection aborted", "Connection refused", "Not connected", "Already connected", "Connection closed", "Initialization error (interapplication manager)", "Bad occurrence", "Wait on unbound occurrence handler", "Occurrence queue overflow", "Datalog type conflict", "Unused", "Unrecognized type (interapplication manager)", "Memory corrupt", "Failed to make temporary DLL", "Old CIN version", "Drag socket not found", "Failed to load drop-object", "Failed to register OLE object", "Failed to release OLE object", "Format specifier type mismatch", "Unknown format specifier", "Too few format specifiers", "Too many format specifiers", "Scan failed", "Newer CIN version", "Error converting to variant", "Runtime menu error", "Password tampered", "Variant attribute not found", "Incompatible variant data type", "Event data is not available", "Event Store is not present", "Occurrence is not found", "Event Queue is not created", "Event info is not available", "Refnum passed is NULL", "Error retrieving Class GUID", "Error retrieving CoClass GUID", "Error retrieving TypeLib GUID.", "Bad built application magic bytes.", "Specific driver is different from the specific driver associated with the Logical Name.", "There is no session opened to the class driver.", "Max Error", "MAX - Error with config objects", "MAX - Error loading configuration", "MAX - Group not supported"]
        # "Handle target error here.\nWhen this JKISM try to communicate with an un-existed JKISM, this JKISM goes into this case."
        # "Handle mistyped state name (developer tool)"
        n58 = Format Into String(format string="Software Exception: Target \"%s\" does not exists." ("message"), error in=w173, w168) -> (resulting string=w176:string, error out=w175:errorcluster)  [unwired: 1 in]
        n59 = call <vilib>:"Error Cluster From Error Code.vi"("show call chain? (False)"=TRUE, "error in (no error)"=w175, "error message (\"\")"=w176, "error code (0)"=w177) -> ("error out"=w174:errorcluster)  [unwired: 5 in]
        n60 = call <vilib>:"Add State(s) to Queue__JKI_lib_State_Machine.vi"("State(s) in (\"\")"=w172) -> ("States Out"=w171:string)  [unwired: 14 in]
      }
      frame "Async Response", "Response" {
        # "Handle Async-call Response (\"Async Response\" for ->)"
        # "Handle Sync-call Response (\"Response\" for @)"
        # "After Message is excuted, JKISM+ goes to this state for recieve the response. \n    For Async Message(->), \"Async Response\" is used. This JKISM will goes to \"Async Message Posted\" immediately and recieve the \"Async Response\" after the callee finishes the message.\n    For Sync Message(@),  This JKISM will wait until the message is done and immidieatly goes to \"Response\""
      }
      frame "Async Message Posted" {
        # "Handle post action for async message (->)."
        # "After Async Message is posted (->), JKISM+ goes to this state for post-action. You can use Argument - State to tell which Async Message is called."
      }
      frame "Initialize Core Data" {
        # "Do not delete, rename, or modify this frame.\n(this is used to determine panel behavior on exit)"
        # "originally closed?"
        # "exe?"
        # "If panel starts closed or is an EXE, then close it when we exit"
        n61 = property class="VI"() -> ("FP.State"=w190:T3)  [unwired: 2 in, 2 out]
        n62 = property class="App"() -> ("App.Kind"=w196:T4)  [unwired: 2 in, 2 out]
        n63 = control-ref of="Current VI Reference"() -> (w191:refnum<vi>)
        n64 = Equal?(x=w190, y=T3."Closed" ("Front Panel Window:State")) -> (x = y?=w188:bool)
        n65 = Equal?(x=w196, y=T4."Run Time System" ("Application:Kind")) -> (x = y?=w194:bool)
        n66 = Or(x=w188, y=w194) -> (x .or. y?=w192:bool)
        n67 = Bundle By Name(cluster=w193, "Core.Current VI Reference"=w191, "Core.Close Panel on Exit?"=w192) -> (w198:T6)
        n68 = call <vilib>:"Add State(s) to Queue__JKI_lib_State_Machine.vi"("State(s) in (\"\")"=w200) -> ("States Out"=w199:string)  [unwired: 14 in]
      }
      frame "Exit" {
        # "Do not put any code in this frame.\n(No errors that occur here will be handled.)"
        n69 = call <vilib>:"Add State(s) to Queue__JKI_lib_State_Machine.vi"("State(s) in (\"\")"=w206) -> ("States Out"=w205:string)  [unwired: 14 in]
      }
      frame "---------- Data ----------" {
        # "Do not put any code in this frame.\n(It is a separator no-op. You can make a copy of this frame to create a new Data frame)"
        n70 = call <vilib>:"Add State(s) to Queue__JKI_lib_State_Machine.vi"("State(s) in (\"\")"=w211) -> ("States Out"=w210:string)  [unwired: 14 in]
      }
      frame "Data: Initialize" {
        w212 = 0  # Transaction Type
        w213 = ""  # Keypad String
        w214 = 0  # New Character
        w216 = T7 {"Current VI Reference"=refnum, "Close Panel on Exit?"=FALSE}  # Core
        w217 = TRUE  # Your Boolean data
        # "Data names and types of shift register data are defined by this bundle."
        # "Initialize the shift-register data, here.\n(data names are defined by what you wire into the bundle function)"
        n71 = Bundle("Core"=w216, "Your Boolean data"=w217, "New Character"=w214, "Keypad String"=w213, "Transaction Type"=w212) -> (w219:T6)  [unwired: 1 in]
        n72 = call <vilib>:"Add State(s) to Queue__JKI_lib_State_Machine.vi"("State(s) in (\"\")"=w221) -> ("States Out"=w220:string)  [unwired: 14 in]
      }
      frame "Data: Cleanup" {
        # "Cleanup any data and references, here.\n(this is called automatically, by the Macro: Exit)"
        n73 = Unbundle By Name(w223) -> ("Core.Current VI Reference"=w226:refnum<vi>)
        n74 = Close Reference(reference=w226, error in (no error)=w225) -> (error out=w224:errorcluster)
        n75 = call <vilib>:"Add State(s) to Queue__JKI_lib_State_Machine.vi"("State(s) in (\"\")"=w228) -> ("States Out"=w227:string)  [unwired: 14 in]
      }
      frame "---------- Events ----------" {
        # "Do not put any code in this frame.\n(It is a separator no-op. You can make a copy of this frame to create a new UI frame)"
        n76 = call <vilib>:"Add State(s) to Queue__JKI_lib_State_Machine.vi"("State(s) in (\"\")"=w233) -> ("States Out"=w232:string)  [unwired: 14 in]
      }
      frame "Events: Register" {
        # "Register message event to break Waiting in Event structure."
        n77 = call <userlib>:"JKISM++ Get New State Notifier Event.vi"("Name(\"\" to use uuid) in"=w236) -> ("Error out"=w234:errorcluster, "New State Notifier Event"=w235:refnum<user-event>)  [unwired: 9 in]
        n78 = register-events(w235) -> (reference out=w237:refnum<event-registration>)  [unwired: 2 in, 1 out]
      }
      frame "Events: Unregister" {
        n79 = Unregister For Events(event registration refnum=w240, error in=w244) -> (error out=w241:errorcluster)
      }
      frame "---------- UI ----------" {
        # "Do not put any code in this frame.\n(It is a separator no-op. You can make a copy of this frame to create a new UI frame)"
        n80 = call <vilib>:"Add State(s) to Queue__JKI_lib_State_Machine.vi"("State(s) in (\"\")"=w249) -> ("States Out"=w248:string)  [unwired: 14 in]
      }
      frame "UI: Initialize" {
        # "Initialize the User Interface, here.\n(this is called automatically, by the Macro: Init)"
        n81 = call <vilib>:"Add State(s) to Queue__JKI_lib_State_Machine.vi"("State(s) in (\"\")"=w254) -> ("States Out"=w253:string)  [unwired: 14 in]
      }
      frame "UI: Cursor Set" {
        # "Argument"
        # "Set and Unset Cursor Busy.\n(Usage: \"UI: Cursor Set >> Busy|Idle\")"
        n82 = case shown="\"Idle\", Default" w256 {
          tunnel: w258 -> [w263 w265]
          tunnel: [w262 w264] -> w257
          frame "Idle", Default {
            n83 = call <vilib>:"Unset Busy.vi"("error in (no error)"=w263) -> ("error out"=w262:errorcluster)  [unwired: 10 in]
          }
          frame "Busy" {
            n84 = call <vilib>:"Set Busy.vi"("error in (no error)"=w265) -> ("error out"=w264:errorcluster)  [unwired: 9 in, 1 out]
          }
        }
        n85 = call <vilib>:"Add State(s) to Queue__JKI_lib_State_Machine.vi"("State(s) in (\"\")"=w261) -> ("States Out"=w260:string)  [unwired: 14 in]
      }
      frame "UI: Front Panel State" {
        # "Argument"
        # "Set Front Panel Open or Closed\n(Usage: \"UI: Front Panel State >> Open|Close\")"
        n86 = Unbundle By Name(w269) -> ("Core.Current VI Reference"=w268:refnum<vi>)
        n87 = case shown="\"Open\", \"Standard\", Default" w267 {
          tunnel: w271 -> [w279 w294 w305 w318 w331]
          tunnel: [w281 w295 w307 w320 w333] -> w270
          tunnel: w268 -> [w280 w292 w306 w319 w332]
          frame "Open", "Standard", Default {
            w274 = T3."Standard" ("State")
            n88 = property class="VI"(reference=w280, error in=w279) -> (reference out=w277:refnum<vi>, error out=w278:errorcluster, "FP.State"=w276:T3)
            n89 = Not Equal?(x=w276, y=w274) -> (x != y?=w275:bool)
            n90 = case shown="False" w275 {
              tunnel: [w285 w287] -> w281
              tunnel: w278 -> [w284 w287]
              tunnel: w277 -> [w283 _]
              tunnel: w274 -> [w282 _]
              frame True {
                n91 = invoke class="VI" method="FP.Open"(reference=w283, error in=w284, "Activate"=TRUE, "State"=w282) -> (error out=w285:errorcluster)  [unwired: 1 in, 4 out]
              }
              frame False {
              }
            }
          }
          frame "Close", "Closed" {
            n92 = property class="VI"(reference=w292, error in=w294) -> (reference out=w291:refnum<vi>, error out=w293:errorcluster, "FP.State"=w289:T3)
            n93 = Not Equal?(x=w289, y=T3."Closed" ("Front Panel Window:State")) -> (x != y?=w288:bool)
            n94 = case shown="True" w288 {
              tunnel: [w296 w299] -> w295
              tunnel: w293 -> [w296 w298]
              tunnel: w291 -> [_ w297]
              frame False {
              }
              frame True {
                n95 = invoke class="VI" method="FP.Close"(reference=w297, error in=w298) -> (error out=w299:errorcluster)  [unwired: 1 in, 2 out]
              }
            }
          }
          frame "Hidden", "Hide" {
            w300 = T3."Hidden" ("State")
            n96 = property class="VI"(reference=w306, error in=w305) -> (reference out=w303:refnum<vi>, error out=w304:errorcluster, "FP.State"=w302:T3)
            n97 = Not Equal?(x=w302, y=w300) -> (x != y?=w301:bool)
            n98 = case shown="True" w301 {
              tunnel: [w311 w312] -> w307
              tunnel: w304 -> [w310 w312]
              tunnel: w303 -> [w309 _]
              tunnel: w300 -> [w308 _]
              frame True {
                n99 = invoke class="VI" method="FP.Open"(reference=w309, error in=w310, "State"=w308) -> (error out=w311:errorcluster)  [unwired: 2 in, 4 out]
              }
              frame False {
              }
            }
          }
          frame "Minimize", "Minimized" {
            w313 = T3."Minimized" ("State")
            n100 = property class="VI"(reference=w319, error in=w318) -> (reference out=w316:refnum<vi>, error out=w317:errorcluster, "FP.State"=w315:T3)
            n101 = Not Equal?(x=w315, y=w313) -> (x != y?=w314:bool)
            n102 = case shown="True" w314 {
              tunnel: [w324 w325] -> w320
              tunnel: w317 -> [w323 w325]
              tunnel: w316 -> [w322 _]
              tunnel: w313 -> [w321 _]
              frame True {
                n103 = invoke class="VI" method="FP.Open"(reference=w322, error in=w323, "State"=w321) -> (error out=w324:errorcluster)  [unwired: 2 in, 4 out]
              }
              frame False {
              }
            }
          }
          frame "Maximize", "Maximized" {
            w326 = T3."Maximized" ("State")
            n104 = property class="VI"(reference=w332, error in=w331) -> (reference out=w329:refnum<vi>, error out=w330:errorcluster, "FP.State"=w328:T3)
            n105 = Not Equal?(x=w328, y=w326) -> (x != y?=w327:bool)
            n106 = case shown="True" w327 {
              tunnel: [w337 w338] -> w333
              tunnel: w330 -> [w336 w338]
              tunnel: w329 -> [w335 _]
              tunnel: w326 -> [w334 _]
              frame True {
                n107 = invoke class="VI" method="FP.Open"(reference=w335, error in=w336, "State"=w334) -> (error out=w337:errorcluster)  [unwired: 2 in, 4 out]
              }
              frame False {
              }
            }
          }
        }
        n108 = call <vilib>:"Add State(s) to Queue__JKI_lib_State_Machine.vi"("State(s) in (\"\")"=w273) -> ("States Out"=w272:string)  [unwired: 14 in]
      }
      frame "---------- Macro ----------" {
        # "Do not put any code in this frame.\n(It is a separator no-op. You can make a copy of this frame to create a new Macro frame)"
        n109 = call <vilib>:"Add State(s) to Queue__JKI_lib_State_Machine.vi"("State(s) in (\"\")"=w343) -> ("States Out"=w342:string)  [unwired: 14 in]
      }
      frame "Macro: Initialize" {
        # "Initialization Macro\n(This is called once, when the VI starts)"
        n110 = call <vilib>:"Add State(s) to Queue__JKI_lib_State_Machine.vi"("State(s) in Front (\"\")"="Data: Initialize\nInitialize Core Data\nEvents: Register\nUI: Initialize\nUI: Front Panel State >> Open\nAction: InitConsole", "State(s) in (\"\")"=w349) -> ("States Out"=w348:string)  [unwired: 13 in]
      }
      frame "Macro: Exit" {
        # "Exit Macro\n(This is called once, when the VI exits)"
        n111 = Unbundle By Name(w357) -> ("Core.Close Panel on Exit?"=w356:bool)
        n112 = Select(t="UI: Front Panel State >> Close", s=w356, f="") -> (s? t:f=w353:string)
        n113 = call <vilib>:"Add State(s) to Queue__JKI_lib_State_Machine.vi"("State(s) in (\"\")"=w353, "State(s) at Back (\"\")"="Action: InitConsole\nData: Cleanup\nEvents: Unregister\nExit") -> ("States Out"=w351:string)  [unwired: 13 in]
        n114 = call <vilib>:"Add State(s) to Queue__JKI_lib_State_Machine.vi"("State(s) in Front (\"\")"=w351, "State(s) in (\"\")"=w360) -> ("States Out"=w359:string)  [unwired: 13 in]
      }
      frame "---------- Action ----------" {
        # "Template Separator\n(You can make a copy of, or modify, this frame)"
        n115 = call <vilib>:"Add State(s) to Queue__JKI_lib_State_Machine.vi"("State(s) in (\"\")"=w365) -> ("States Out"=w364:string)  [unwired: 14 in]
      }
      frame "Action: InitConsole" {
        # "Template Separator\n(You can make a copy of, or modify, this frame)"
        n116 = property on="Transactions" class="Clust"(error in=w367, "DisabledEnum"=T5."Disabled and Grayed Out" ("Disabled")) -> (error out=w371:errorcluster)  [unwired: 1 in, 1 out]
        n117 = property on="Card Reader" class="Bool (strict)"(error in=w367, "DisabledEnum"=T5."Enabled" ("Disabled")) -> (error out=w370:errorcluster)  [unwired: 1 in, 1 out]
        n118 = property on="Keypad" class="Clust"(error in=w367, "DisabledEnum"=T5."Disabled and Grayed Out" ("Disabled")) -> (error out=w366:errorcluster)  [unwired: 1 in, 1 out]
        n119 = Merge Errors(w371, w366, w370) -> (w369:errorcluster)
        n120 = call <vilib>:"Add State(s) to Queue__JKI_lib_State_Machine.vi"("State(s) in (\"\")"=w377) -> ("States Out"=w376:string)  [unwired: 14 in]
      }
      frame "Action: PostErr" {
        # "Copy/Rename this case for your own API"
        n121 = call <userlib>:"JKISM++ Check If Module Exists.vi"("Error in"=w380, "JKISM Name"="Error Handler" ("Dest Module (\"\")")) -> ("Error out"=w379:errorcluster, "Exist?"=w382:bool)  [unwired: 7 in, 1 out]
        n122 = case shown="False" w382 {
          tunnel: w381 -> [_ w396]
          tunnel: ["Macro: Exit" w389] -> w378
          frame False {
          }
          frame True {
            n123 = call <userlib>:"Build State String with Arguments++.vi"("State"="Error Handler", "Arguments (\"\")"=w396, "Dest Module (\"\")"="Error Handler" ("Dest Module (\"\")"), "Sync-Call(@) T By Default/Async-Call(->) F"=FALSE) -> ("State with Arguments"=w390:string)  [unwired: 11 in]
            n124 = Concatenate Strings(w390, "\r", "Macro: Exit") -> (w389:string)
          }
        }
        n125 = call <vilib>:"Add State(s) to Queue__JKI_lib_State_Machine.vi"("State(s) in (\"\")"=w385, "State(s) at Back (\"\")"=w378) -> ("States Out"=w384:string)  [unwired: 13 in]
      }
      frame "Action: Card Reader" {
        # "Copy/Rename this case for your own API"
        n126 = call <userlib>:"JKISM++ Convert Data to HexStr.vi"("Variant"=TRUE) -> ("HEX String (0-9,A-F)"=w410:string)  [unwired: 8 in]
        n127 = call <userlib>:"Build State String with Arguments++.vi"("State"="Action: Log In Init" ("States"), "Arguments (\"\")"="John,Doe" ("Arguments (\"\")"), "Dest Module (\"\")"="Controller" ("Dest Module"), "Sync-Call(@) T By Default/Async-Call(->) F"=FALSE) -> ("State with Arguments"=w404:string)  [unwired: 11 in]
        n128 = call <userlib>:"Build State String with Arguments++.vi"("State"="Action: Card" ("States"), "Arguments (\"\")"=w410, "Dest Module (\"\")"="Display" ("Dest Module"), "Sync-Call(@) T By Default/Async-Call(->) F"=FALSE) -> ("State with Arguments"=w405:string)  [unwired: 11 in]
        n129 = Concatenate Strings(w405, "\r", w404) -> (w399:string)
        n130 = call <vilib>:"Add State(s) to Queue__JKI_lib_State_Machine.vi"("State(s) in (\"\")"=w401, "State(s) at Back (\"\")"=w399) -> ("States Out"=w400:string)  [unwired: 13 in]
      }
      frame "Action: Keypad" {
        # "Do not put any code in this frame.\n(It is a separator no-op. This category is recommanded to use for external API)"
        n131 = Unbundle By Name(w417) -> ("Keypad String"=w423:string)
        n132 = Bundle By Name(cluster=w417, "Keypad String"="") -> (w415:T6)
        n133 = call <userlib>:"Build State String with Arguments++.vi"("State"="Action: Receive Keypad" ("States"), "Arguments (\"\")"=w423, "Dest Module (\"\")"="Controller" ("Dest Module"), "Sync-Call(@) T By Default/Async-Call(->) F"=FALSE) -> ("State with Arguments"=w418:string)  [unwired: 11 in]
        n134 = call <vilib>:"Add State(s) to Queue__JKI_lib_State_Machine.vi"("State(s) in (\"\")"=w420, "State(s) at Back (\"\")"=w418) -> ("States Out"=w419:string)  [unwired: 13 in]
      }
      frame "Action: Transaction" {
        # "Do not put any code in this frame.\n(It is a separator no-op. This category is recommanded to use for external API)"
        n135 = Unbundle By Name(w432) -> ("Transaction Type"=w431:i32)
        n136 = case shown="2" w431 {
          tunnel: [w435 w439 w443 w446 w451 w454 w459 _] -> w428
          frame 0 {
            n137 = call <userlib>:"Build State String with Arguments++.vi"("State"="Action: Balance" ("States"), "Dest Module (\"\")"="Controller" ("Dest Module"), "Sync-Call(@) T By Default/Async-Call(->) F"=FALSE) -> ("State with Arguments"=w435:string)  [unwired: 12 in]
          }
          frame 1 {
            n138 = call <userlib>:"Build State String with Arguments++.vi"("State"="Action: Deposit Init" ("States"), "Dest Module (\"\")"="Controller" ("Dest Module"), "Sync-Call(@) T By Default/Async-Call(->) F"=FALSE) -> ("State with Arguments"=w439:string)  [unwired: 12 in]
          }
          frame 2 {
            n139 = call <userlib>:"Build State String with Arguments++.vi"("State"="Action: Withdraw Init" ("States"), "Dest Module (\"\")"="Controller" ("Dest Module"), "Sync-Call(@) T By Default/Async-Call(->) F"=FALSE) -> ("State with Arguments"=w443:string)  [unwired: 12 in]
          }
          frame 3 {
            n140 = call <userlib>:"Build State String with Arguments++.vi"("State"="Action: Fast Cash Enough" ("States"), "Dest Module (\"\")"="Controller" ("Dest Module"), "Sync-Call(@) T By Default/Async-Call(->) F"=FALSE) -> ("State with Arguments"=w446:string)  [unwired: 12 in]
          }
          frame 4 {
            n141 = call <userlib>:"Build State String with Arguments++.vi"("State"="Action: New Transaction" ("States"), "Dest Module (\"\")"="Controller" ("Dest Module"), "Sync-Call(@) T By Default/Async-Call(->) F"=FALSE) -> ("State with Arguments"=w451:string)  [unwired: 12 in]
          }
          frame 5 {
            n142 = call <userlib>:"Build State String with Arguments++.vi"("State"="Action: Cancel Transaction" ("States"), "Dest Module (\"\")"="Controller" ("Dest Module"), "Sync-Call(@) T By Default/Async-Call(->) F"=FALSE) -> ("State with Arguments"=w454:string)  [unwired: 12 in]
          }
          frame 6 {
            n143 = call <userlib>:"Build State String with Arguments++.vi"("State"="Action: Terminate" ("States"), "Dest Module (\"\")"="Controller" ("Dest Module"), "Sync-Call(@) T By Default/Async-Call(->) F"=FALSE) -> ("State with Arguments"=w459:string)  [unwired: 12 in]
          }
          frame Default {
          }
        }
        n144 = call <vilib>:"Add State(s) to Queue__JKI_lib_State_Machine.vi"("State(s) in (\"\")"=w430, "State(s) at Back (\"\")"=w428) -> ("States Out"=w429:string)  [unwired: 13 in]
      }
      frame "Action: Keypad String" {
        # "1...12"
        # "Template Separator\n(You can make a copy of, or modify, this frame)"
        n145 = Unbundle By Name(w465) -> ("Keypad String"=w466:string, "New Character"=w467:i32)
        n146 = case shown="12" w467 {
          selector: w467 -> [_ w475 _ _ _]
          tunnel: w466 -> [_ w472 w476 w479 w483]
          tunnel: [_ w473 w477 w480 w483] -> w462
          tunnel: [_ _ _ _ "Action: KeyPad" ("States")] -> w463
          frame 0, Default {
          }
          frame 1..9 {
            n147 = Number To Decimal String(number=w475) -> (decimal integer string=w474:string)  [unwired: 1 in]
            n148 = Concatenate Strings(w472, w474) -> (w473:string)
          }
          frame 10 {
            n149 = Concatenate Strings(w476, "0" ("string")) -> (w477:string)
          }
          frame 11 {
            n150 = String Length(string=w479) -> (length=w482:i32)
            n151 = Decrement(x=w482) -> (x-1=w481:i32)
            n152 = String Subset(string=w479, length (rest)=w481) -> (substring=w480:string)  [unwired: 1 in]
          }
          frame 12 {
          }
        }
        "Keypad String" <- w462
        n153 = Bundle By Name(cluster=w465, "Keypad String"=w462) -> (w464:T6)
        n154 = call <vilib>:"Add State(s) to Queue__JKI_lib_State_Machine.vi"("State(s) in Front (\"\")"=w463, "State(s) in (\"\")"=w471) -> ("States Out"=w470:string)  [unwired: 13 in]
      }
      frame "Action: Enable Card Reader" {
        # "Your code here.\n(You can make a copy of, or modify, this frame)"
        n155 = property on="Card Reader" class="Bool (strict)"(error in=w486, "DisabledEnum"=T5."Enabled" ("Disabled")) -> (error out=w485:errorcluster)  [unwired: 1 in, 1 out]
        n156 = call <vilib>:"Add State(s) to Queue__JKI_lib_State_Machine.vi"("State(s) in (\"\")"=w491) -> ("States Out"=w490:string)  [unwired: 14 in]
      }
      frame "Action: Enable Keypad" {
        # "Your code here.\n(You can make a copy of, or modify, this frame)"
        n157 = property on="Keypad" class="Clust"(error in=w493, "DisabledEnum"=T5."Enabled" ("Disabled")) -> (error out=w492:errorcluster)  [unwired: 1 in, 1 out]
        n158 = call <vilib>:"Add State(s) to Queue__JKI_lib_State_Machine.vi"("State(s) in (\"\")"=w498) -> ("States Out"=w497:string)  [unwired: 14 in]
      }
      frame "Action: Enable Transaction" {
        # "Template Separator\n(You can make a copy of, or modify, this frame)"
        n159 = property on="Transactions" class="Clust"(error in=w500, "DisabledEnum"=T5."Enabled" ("Disabled")) -> (error out=w499:errorcluster)  [unwired: 1 in, 1 out]
        n160 = call <vilib>:"Add State(s) to Queue__JKI_lib_State_Machine.vi"("State(s) in (\"\")"=w505) -> ("States Out"=w504:string)  [unwired: 14 in]
      }
      frame "Action: Disable Card Reader" {
        # "Template Separator\n(You can make a copy of, or modify, this frame)"
        n161 = property on="Card Reader" class="Bool (strict)"(error in=w507, "DisabledEnum"=T5."Disabled and Grayed Out" ("Disabled")) -> (error out=w506:errorcluster)  [unwired: 1 in, 1 out]
        n162 = call <vilib>:"Add State(s) to Queue__JKI_lib_State_Machine.vi"("State(s) in (\"\")"=w512) -> ("States Out"=w511:string)  [unwired: 14 in]
      }
      frame "Action: Disable Keypad" {
        # "Template Separator\n(You can make a copy of, or modify, this frame)"
        n163 = property on="Keypad" class="Clust"(error in=w514, "DisabledEnum"=T5."Disabled and Grayed Out" ("Disabled")) -> (error out=w513:errorcluster)  [unwired: 1 in, 1 out]
        n164 = call <vilib>:"Add State(s) to Queue__JKI_lib_State_Machine.vi"("State(s) in (\"\")"=w519) -> ("States Out"=w518:string)  [unwired: 14 in]
      }
      frame "Action: Disable Transaction" {
        # "Template Separator\n(You can make a copy of, or modify, this frame)"
        n165 = property on="Transactions" class="Clust"(error in=w521, "DisabledEnum"=T5."Disabled and Grayed Out" ("Disabled")) -> (error out=w520:errorcluster)  [unwired: 1 in, 1 out]
        n166 = call <vilib>:"Add State(s) to Queue__JKI_lib_State_Machine.vi"("State(s) in (\"\")"=w526) -> ("States Out"=w525:string)  [unwired: 14 in]
      }
    }
  }
